vi "GUI_Bella_2BLMap.vi"() -> ()   [LabVIEW 2020]
uses:
  Shared/GUI_Template/GUI_master/tcp_new_data_event.ctl
  Shared/GUI_Template/GUI_master/tcp new data cluster.ctl
panel:
  in  "pos.Channel0::7":enum16{"1", "2", "3", "4", "5", "6"}(ring) caption="F3M5 FW"
  in  "Position::6":dbl caption="F3M3 Iris" min=-50.0 max=50.0 format="%#_6p"
  in  "Position::4":dbl caption="M3A Iris" min=-50.0 max=50.0 format="%#_6p"
  in  "pos.Channel0::9":enum16{"1", "2", "3", "4", "5", "6"}(ring) caption="Ghost FW"
  in  "pos.Channel0::8":enum16{"1", "2", "3", "4", "5", "6"}(ring) caption="F3M7 FW"
  in  "pos.Channel0::3":enum16{"1", "2", "3", "4", "5", "6"}(ring) caption="M2A FW"
  in  "pos.Channel3::1":enum16{"1", "2", "3", "4", "5", "6"}(ring) caption="SPLIT FW"
  in  "GUIdevice 9":string="FW-PL1-GHOST"
  in  "GUIdevice 8":string="FW"
  in  "GUIdevice 7":string="FW"
  in  "GUIdevice 6":string="IRIS-2BL-F3M3"
  in  "GUIdevice 5":string="IRIS"
  in  "GUIdevice 4":string="IRIS-2BL-M3A"
  in  "GUIdevice 3":string="FW-2BL-M2A"
  in  "GUIdevice 2":string="IRIS"
  in  "GUIdevice 1":string="FW-LT-DM"
  in  "Ghost Cam":bool caption="HPDCCD2"
  in  "F3M7 Cam":bool caption="HPDCCD2"
  in  "F3M5 Cam":bool caption="HPDCCD2"
  in  "F3M3 Cam":bool caption="HPDCCD2"
  in  "M4A Cam":bool caption="HPDCCD2"
  in  "M3A Cam":bool
  in  "M2A Cam":bool caption="HPDCCD2"
  in  "2BL DM Cam":bool caption="HPDCCD2"
  in  "SPLIT Cam":bool caption="HPDCCD2"
  out "tcp data event":T1
  in  "stop":bool
  out "error IO 2":errorcluster
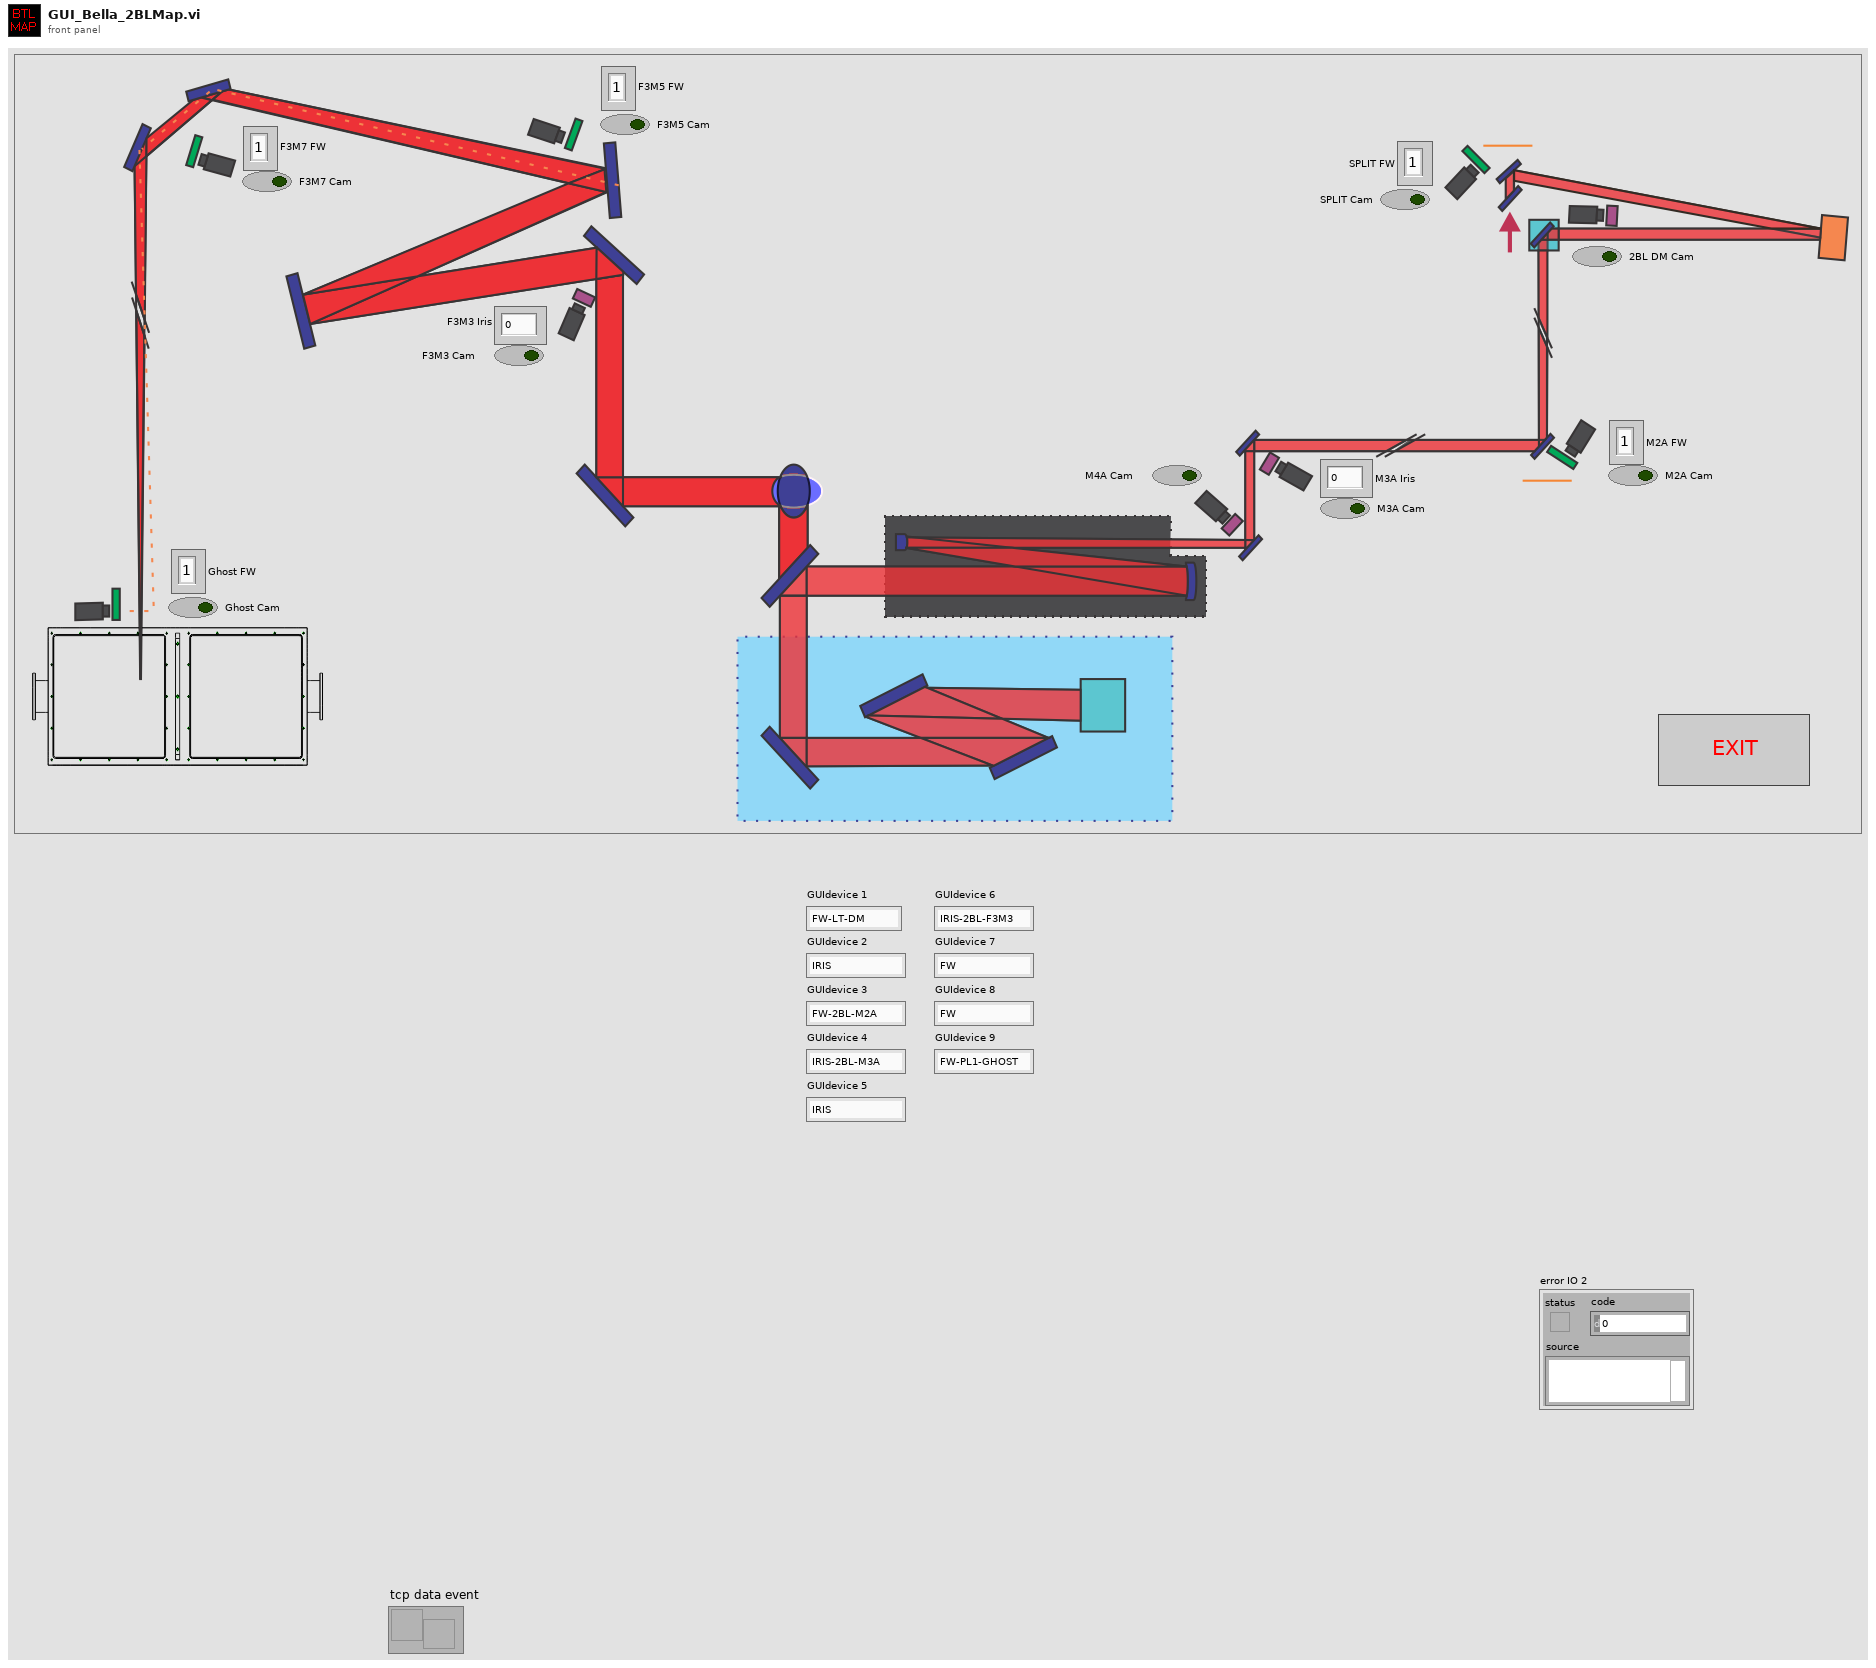
[diagram p1: front panel]
types:
  T1 = typedef "tcp_new_data_event.ctl" = refnum<user-event>
  T2 = typedef "tcp new data cluster.ctl" = cluster{"EventEnum":enum16{"new data", "connection status update"}, "Device name":string}
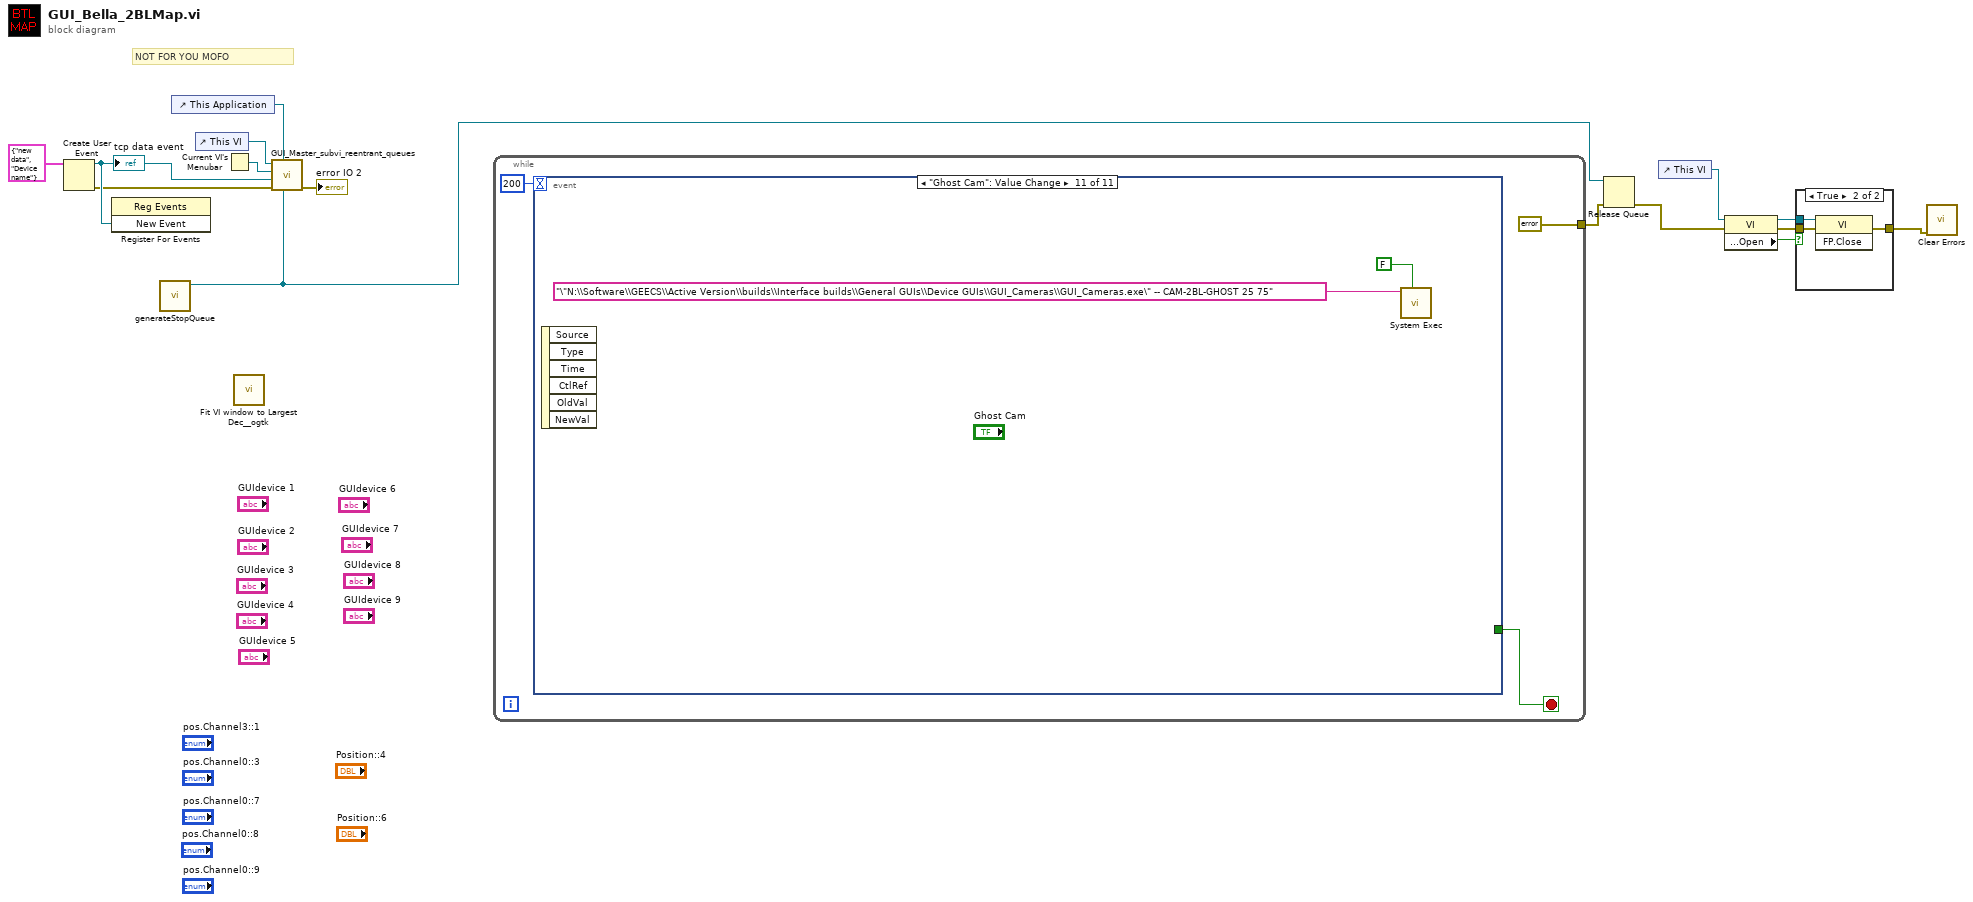
[diagram p0: block diagram]
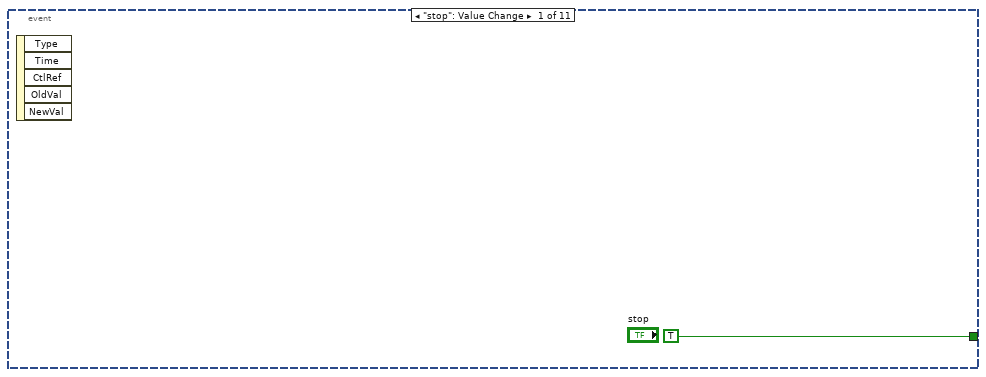
[diagram p3: hidden frame]
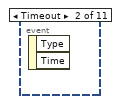
[diagram p4: hidden frame]
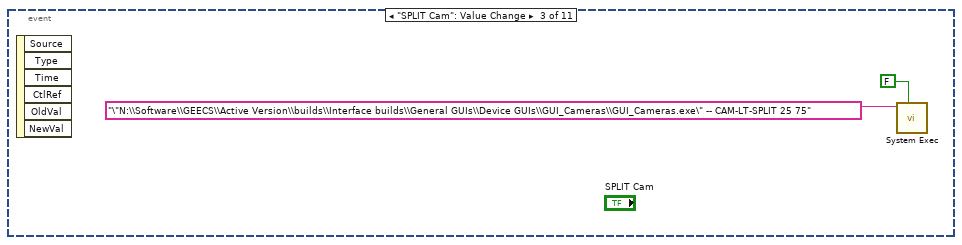
[diagram p5: hidden frame]
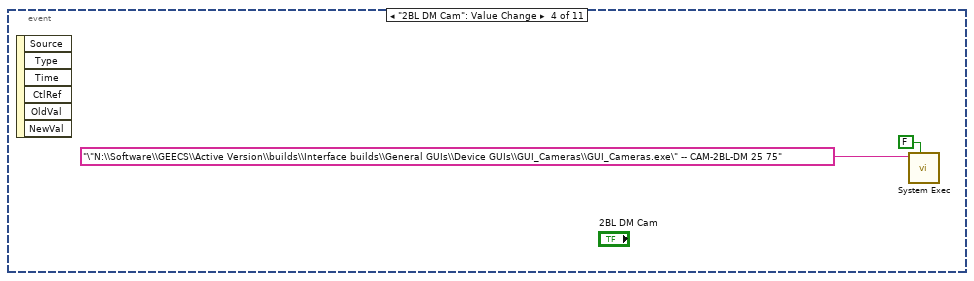
[diagram p6: hidden frame]
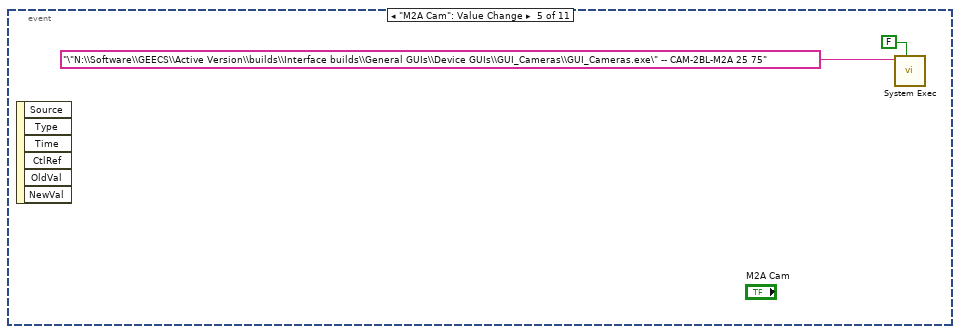
[diagram p7: hidden frame]
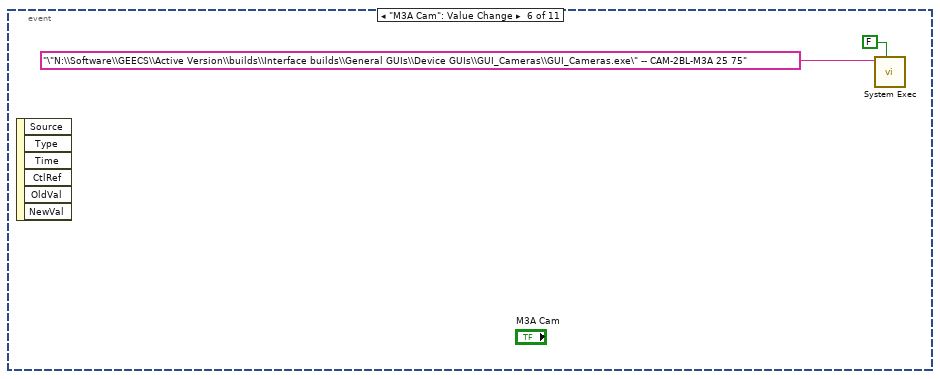
[diagram p8: hidden frame]
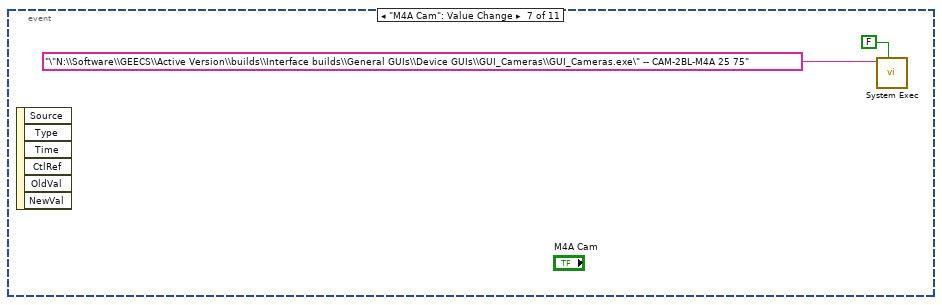
[diagram p9: hidden frame]
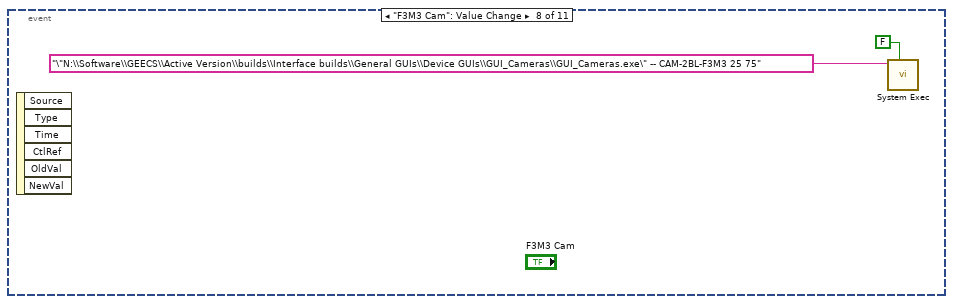
[diagram p10: hidden frame]
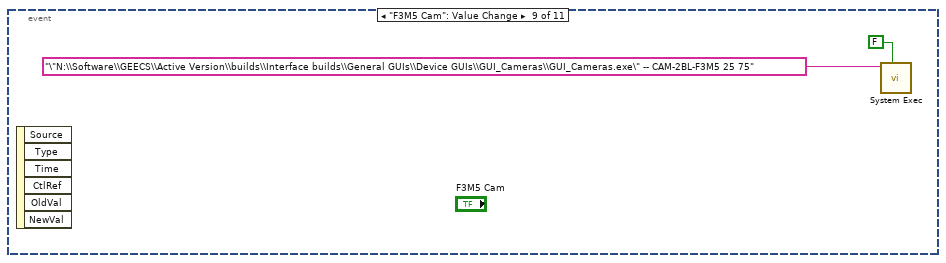
[diagram p11: hidden frame]
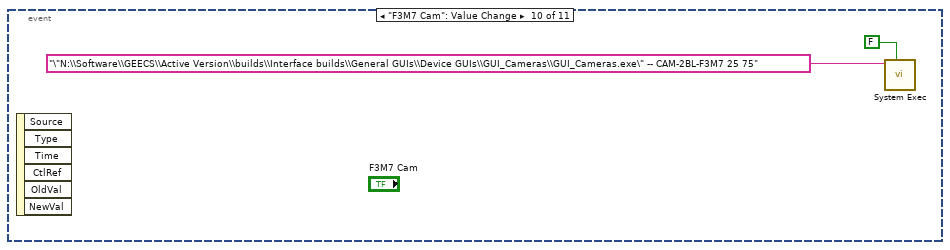
[diagram p12: hidden frame]
diagram:
  # "NOT FOR YOU MOFO"
  n1 = Create User Event(user event datatype=T2 {"EventEnum"=enum."new data", "Device name"="Device name"} ("New Event")) -> (user event=w14:refnum<user-event>, error out=w13:errorcluster)  [unwired: 1 in]
  "tcp data event" <- w14
  n2 = register-events(w14) -> ()  [unwired: 2 in, 2 out]
  n3 = call "generateStopQueue.vi"() -> ("STOP Queue out"=w8:refnum<queue>)  [unwired: 10 in, 1 out]
  n4 = control-ref of="This Application"() -> (w15:refnum<vi>)
  n5 = control-ref of="This VI"() -> (w10:refnum<vi>)
  n6 = Current VI's Menubar() -> (w11:refnum<k9>)
  n7 = call <userlib>:"Fit VI window to Largest Dec__ogtk.vi"() -> ()  [unwired: 6 in, 2 out]
  n8 = call "GUI_Master_subvi_reentrant_queues.vi"("STOP Queue in"=w8, "This Application"=w15, "error in (no error)"=w13, "tcp data event"=w14, "Caller menu reference"=w11, "Caller VI ref"=w10) -> ("error out"=→"error IO 2":errorcluster)  [unwired: 5 in]
  n9 = while {
    tunnel: [errorcluster {"status"=FALSE, "code"=0, "source"=""} ("error in (no error)")] -> w7
    stop <- w18 stop-if-true
    n10 = event shown="[10] \"Ghost Cam\": Value Change" {
      selector: _ -> [_ _ _ _ _ _ _ _ _ _ _]
      dyn-events: _ -> [_ _ _ _ _ _ _ _ _ _ _]
      timeout: 200 -> [_ _ _ _ _ _ _ _ _ _ _]
      tunnel: [TRUE ("stop") _ _ _ _ _ _ _ _ _ _] -> w18
      event "stop": Value Change {
        n11 = event-data() -> ()  [unwired: 1 in, 5 out]
      }
      event Timeout {
        n12 = event-data() -> ()  [unwired: 1 in, 2 out]
      }
      event "SPLIT Cam": Value Change {
        n13 = event-data() -> ()  [unwired: 1 in, 6 out]
        n14 = call <vilib>:"System Exec.vi"("wait until completion? (T)"=FALSE, "command line"="\"N:\\Software\\GEECS\\Active Version\\builds\\Interface builds\\General GUIs\\Device GUIs\\GUI_Cameras\\GUI_Cameras.exe\" -- CAM-LT-SPLIT 25 75") -> ()  [unwired: 6 in, 4 out]
      }
      event "2BL DM Cam": Value Change {
        n15 = event-data() -> ()  [unwired: 1 in, 6 out]
        n16 = call <vilib>:"System Exec.vi"("wait until completion? (T)"=FALSE, "command line"="\"N:\\Software\\GEECS\\Active Version\\builds\\Interface builds\\General GUIs\\Device GUIs\\GUI_Cameras\\GUI_Cameras.exe\" -- CAM-2BL-DM 25 75") -> ()  [unwired: 6 in, 4 out]
      }
      event "M2A Cam": Value Change {
        n17 = event-data() -> ()  [unwired: 1 in, 6 out]
        n18 = call <vilib>:"System Exec.vi"("wait until completion? (T)"=FALSE, "command line"="\"N:\\Software\\GEECS\\Active Version\\builds\\Interface builds\\General GUIs\\Device GUIs\\GUI_Cameras\\GUI_Cameras.exe\" -- CAM-2BL-M2A 25 75") -> ()  [unwired: 6 in, 4 out]
      }
      event "M3A Cam": Value Change {
        n19 = event-data() -> ()  [unwired: 1 in, 6 out]
        n20 = call <vilib>:"System Exec.vi"("wait until completion? (T)"=FALSE, "command line"="\"N:\\Software\\GEECS\\Active Version\\builds\\Interface builds\\General GUIs\\Device GUIs\\GUI_Cameras\\GUI_Cameras.exe\" -- CAM-2BL-M3A 25 75") -> ()  [unwired: 6 in, 4 out]
      }
      event "M4A Cam": Value Change {
        n21 = event-data() -> ()  [unwired: 1 in, 6 out]
        n22 = call <vilib>:"System Exec.vi"("wait until completion? (T)"=FALSE, "command line"="\"N:\\Software\\GEECS\\Active Version\\builds\\Interface builds\\General GUIs\\Device GUIs\\GUI_Cameras\\GUI_Cameras.exe\" -- CAM-2BL-M4A 25 75") -> ()  [unwired: 6 in, 4 out]
      }
      event "F3M3 Cam": Value Change {
        n23 = event-data() -> ()  [unwired: 1 in, 6 out]
        n24 = call <vilib>:"System Exec.vi"("wait until completion? (T)"=FALSE, "command line"="\"N:\\Software\\GEECS\\Active Version\\builds\\Interface builds\\General GUIs\\Device GUIs\\GUI_Cameras\\GUI_Cameras.exe\" -- CAM-2BL-F3M3 25 75") -> ()  [unwired: 6 in, 4 out]
      }
      event "F3M5 Cam": Value Change {
        n25 = event-data() -> ()  [unwired: 1 in, 6 out]
        n26 = call <vilib>:"System Exec.vi"("wait until completion? (T)"=FALSE, "command line"="\"N:\\Software\\GEECS\\Active Version\\builds\\Interface builds\\General GUIs\\Device GUIs\\GUI_Cameras\\GUI_Cameras.exe\" -- CAM-2BL-F3M5 25 75") -> ()  [unwired: 6 in, 4 out]
      }
      event "F3M7 Cam": Value Change {
        n27 = event-data() -> ()  [unwired: 1 in, 6 out]
        n28 = call <vilib>:"System Exec.vi"("wait until completion? (T)"=FALSE, "command line"="\"N:\\Software\\GEECS\\Active Version\\builds\\Interface builds\\General GUIs\\Device GUIs\\GUI_Cameras\\GUI_Cameras.exe\" -- CAM-2BL-F3M7 25 75") -> ()  [unwired: 6 in, 4 out]
      }
      event "Ghost Cam": Value Change {
        n29 = event-data() -> ()  [unwired: 1 in, 6 out]
        n30 = call <vilib>:"System Exec.vi"("wait until completion? (T)"=FALSE, "command line"="\"N:\\Software\\GEECS\\Active Version\\builds\\Interface builds\\General GUIs\\Device GUIs\\GUI_Cameras\\GUI_Cameras.exe\" -- CAM-2BL-GHOST 25 75") -> ()  [unwired: 6 in, 4 out]
      }
    }
  }
  n31 = Release Queue(queue=w8, error in (no error)=w7) -> (error out=w2:errorcluster)  [unwired: 1 in, 2 out]
  n32 = control-ref of="This VI"() -> (w3:refnum<vi>)
  n33 = property class="VI"(reference=w3, error in=w2) -> (reference out=w5:refnum<vi>, error out=w6:errorcluster, "Front Panel.Open"=w4:bool)
  n34 = case shown="True" w4 {
    tunnel: [w38 w41] -> w1
    tunnel: w6 -> [w38 w40]
    tunnel: w5 -> [_ w39]
    frame False {
    }
    frame True {
      n35 = invoke class="VI" method="FP.Close"(reference=w39, error in=w40) -> (error out=w41:errorcluster)  [unwired: 1 in, 2 out]
    }
  }
  n36 = call <vilib>:"Clear Errors.vi"("error in (no error)"=w1) -> ()  [unwired: 5 in, 2 out]
